vi "Route.vi"(8 "error in (no error)":errorcluster, 9 "Connect":bool, 10 "channel 1":string caption="Route", 11 "reference in":refnum<class "SwitchBase.lvclass">) -> (0 "error out":errorcluster, 3 "reference in":refnum<class "SwitchBase.lvclass">)   [LabVIEW 2022 SP3, in "SwitchBase.lvlib" / "SwitchBase.lvclass"]
uses:
  SwitchBase.lvclass
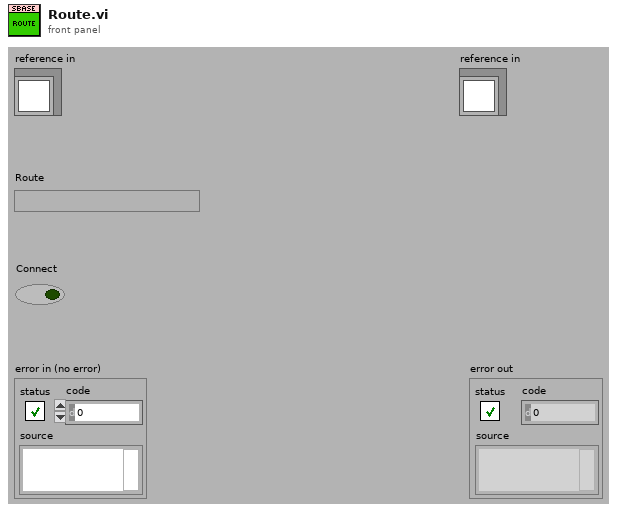
[diagram p1: front panel]
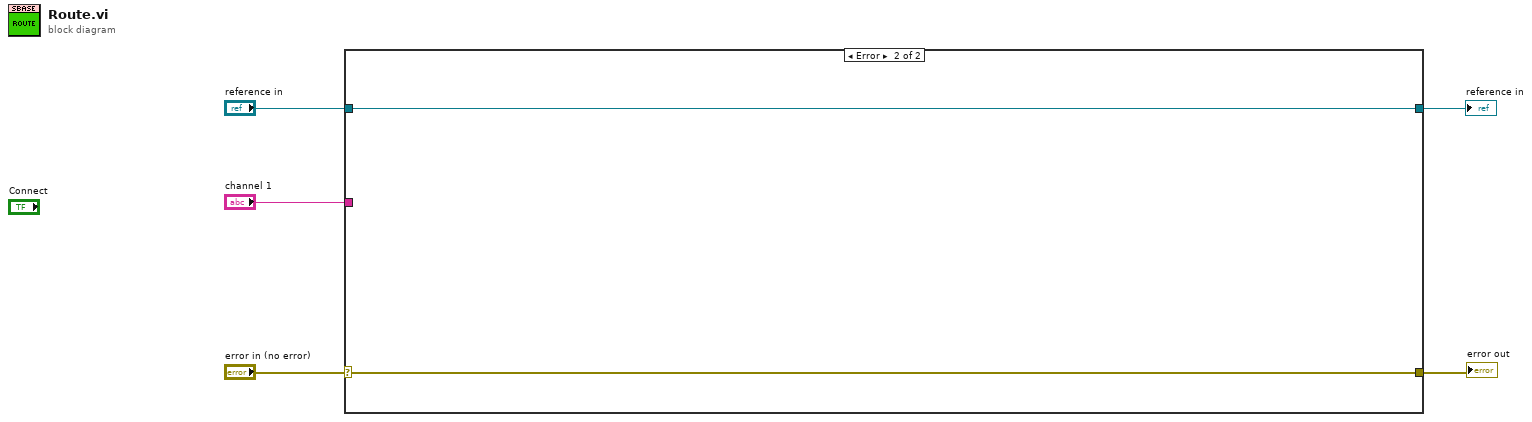
[diagram p0: block diagram]
diagram:
  n1 = case shown="Error" "error in (no error)" {
    selector: "error in (no error)" -> [w7 w9]
    tunnel: [w7 w9] -> w4
    tunnel: [w6 w8] -> w2
    tunnel: "reference in" -> [w6 w8]
    tunnel: "channel 1" -> [_ _]
    frame No Error {
    }
    frame Error {
    }
  }
  "error out" <- w4
  "reference in" <- w2
